vi "svx_Continuous Broadband Waveform.vi"(5 "signal type":T1(ring)=enum."Uniform white noise", 6 "sampling info":cluster{"Fs":dbl, "#s":dbl}={"Fs"=1000.0, "#s"=1000.0} {"Fs" format="%.2p"}, 7 "generation control":T2(ring), 8 "error in":errorcluster, 9 "delay until transition (0 samples)":i32, 10 "initial waveform state":cluster{"amplitude":dbl, "offset":dbl, "tf":dbl} {"tf" format="%.2f"; "offset" format="%.2f"; "amplitude" format="%.2f"}, 11 "desired waveform state":T3={"amplitude"=1.0, "offset"=0.0, "tf (ignored)"=0.0} {"tf (ignored)" format="%.2f"; "offset" format="%.2p"; "amplitude" format="%.2p"}) -> (0 "error out":errorcluster, 1 "index of transition":i32, 2 "final waveform state":cluster{"amplitude":dbl, "offset":dbl, "tf":dbl} {"tf" format="%.2f"; "offset" format="%.2f"; "amplitude" format="%.2f"}, 3 "signal out":waveform(dbl))   [LabVIEW 2017]
uses:
  <vilib>/Analysis/baseanly.llb/Inverse f Filter (DBL).vi
  <vilib>/Analysis/NI_AALBase.lvlib
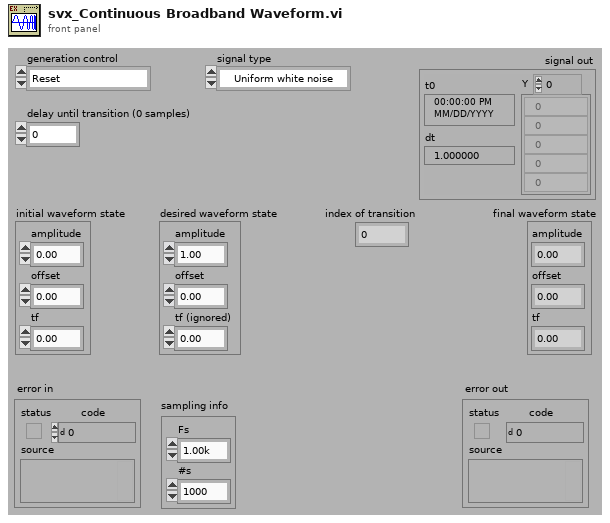
[diagram p1: front panel]
types:
  T1 = enum16{"Sine wave", "Dual tone (IMD)", "Multitone", "Chirp", "Frequency flat chirp", "Uniform white noise", "Gaussian white noise", "Pink noise", "PRN"}
  T2 = enum16{"Reset", "Continue from previous", "Continue from state", "Zero from previous", "Zero from state"}
  T3 = cluster{"amplitude":dbl, "offset":dbl, "tf (ignored)":dbl}
  T4 = cluster{"lower cutoff freq":dbl, dbl, "order":i32}
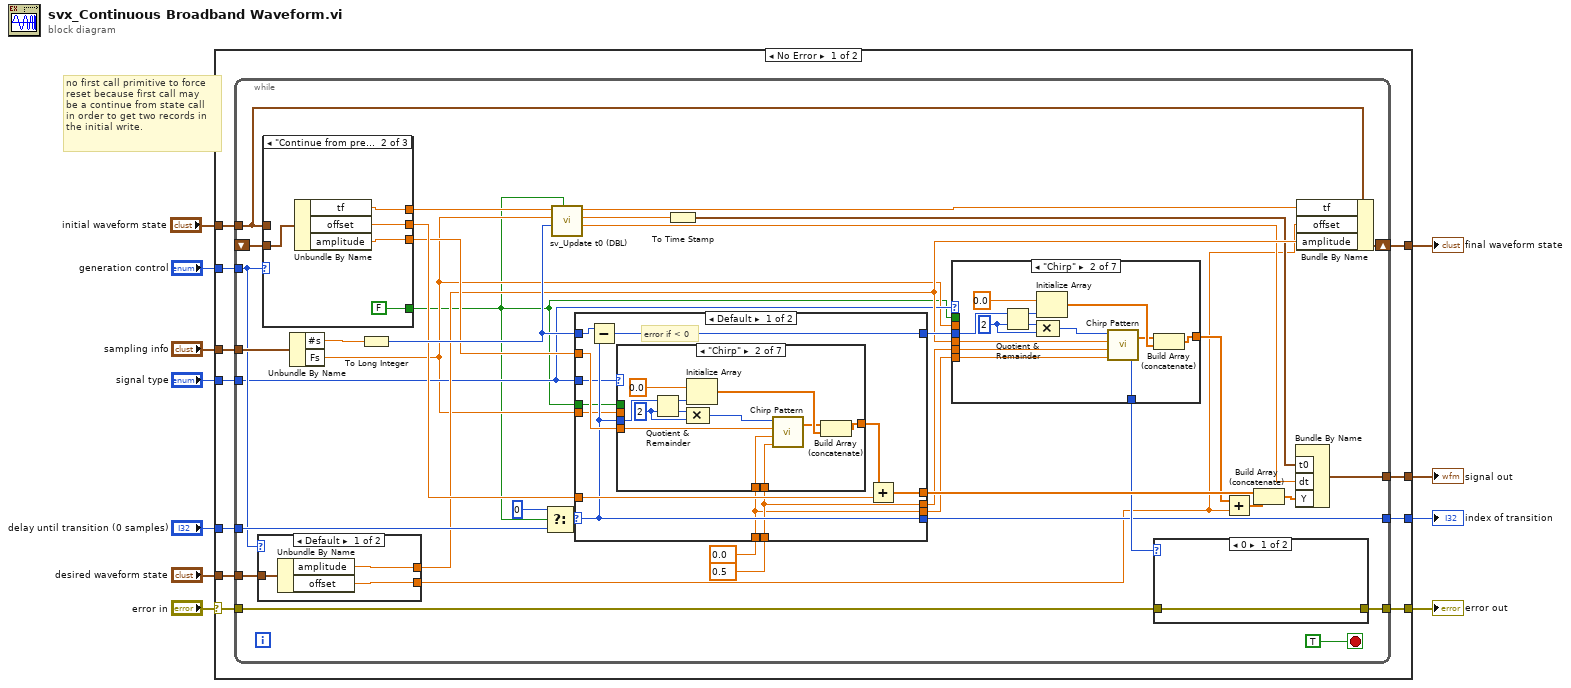
[diagram p0: block diagram]
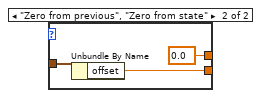
[diagram p2: hidden frame]
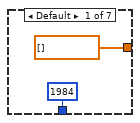
[diagram p3: hidden frame]
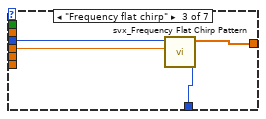
[diagram p4: hidden frame]
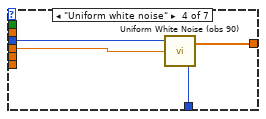
[diagram p5: hidden frame]
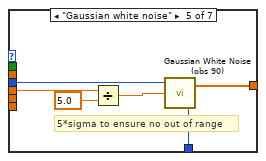
[diagram p6: hidden frame]
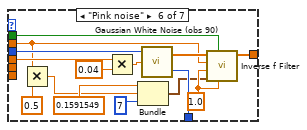
[diagram p7: hidden frame]
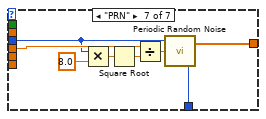
[diagram p8: hidden frame]
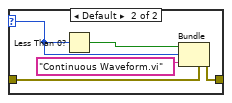
[diagram p9: hidden frame]
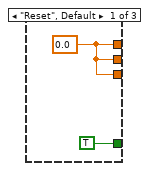
[diagram p10: hidden frame]
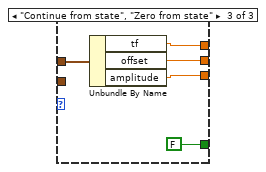
[diagram p11: hidden frame]
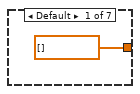
[diagram p12: hidden frame]
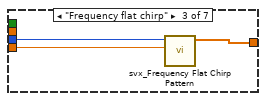
[diagram p13: hidden frame]
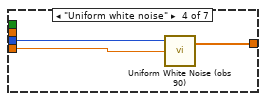
[diagram p14: hidden frame]
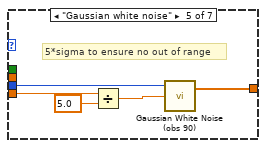
[diagram p15: hidden frame]
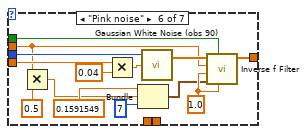
[diagram p16: hidden frame]
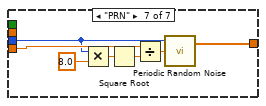
[diagram p17: hidden frame]
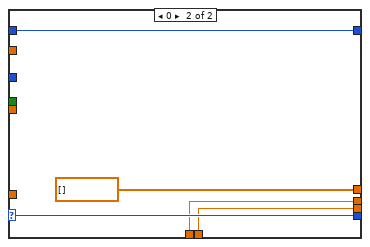
[diagram p18: hidden frame]
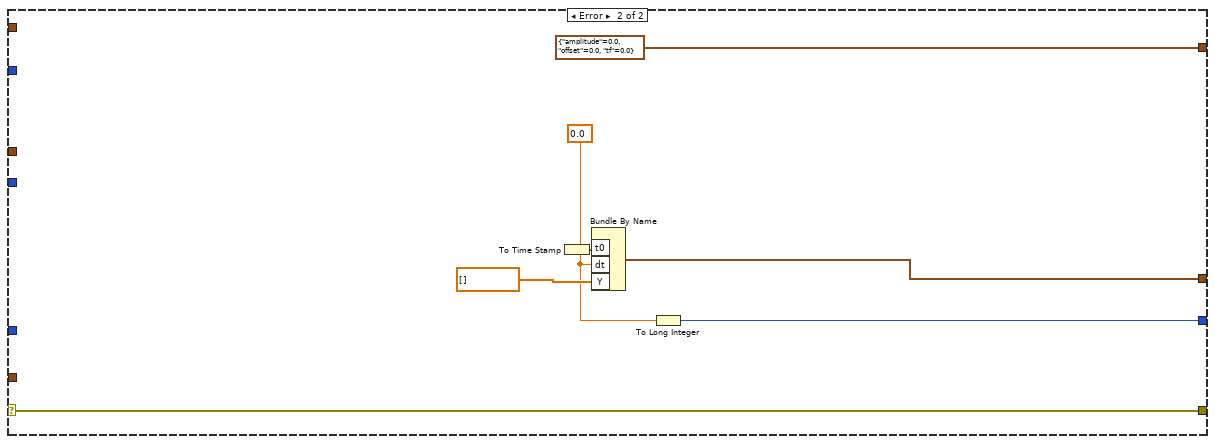
[diagram p19: hidden frame]
diagram:
  # "no first call primitive to force \nreset because first call may \nbe a continue from state call\nin order to get two records in \nthe initial write."
  n1 = case shown="No Error" "error in" {
    selector: "error in" -> [w19 w204]
    tunnel: [w21 w204] -> w10
    tunnel: [w20 w205] -> w1
    tunnel: [w18 w201] -> w9
    tunnel: "delay until transition (0 samples)" -> [w17 _]
    tunnel: [w16 cluster{"amplitude":dbl, "offset":dbl, "tf":dbl} {"amplitude"=0.0, "offset"=0.0, "tf"=0.0} ("initial waveform state")] -> w7
    tunnel: "generation control" -> [w15 _]
    tunnel: "desired waveform state" -> [w14 _]
    tunnel: "initial waveform state" -> [w13 _]
    tunnel: "signal type" -> [w12 _]
    tunnel: "sampling info" -> [w22 _]
    frame No Error {
      n2 = while {
        tunnel: w13 -> [w47]
        tunnel: w14 -> [w49]
        tunnel: w15 -> [w35]
        shift-left: _ -> [w53]
        shift-right: [w42] -> w16
        tunnel: w17 -> [w39]
        tunnel: [w31] -> w18
        tunnel: w19 -> [w45]
        tunnel: [w58] -> w20
        tunnel: [w44] -> w21
        tunnel: w12 -> [w33]
        tunnel: w22 -> [w59]
        stop <- TRUE stop-if-true
        n3 = case shown="Default" w35 {
          tunnel: w49 -> [w63 w65]
          tunnel: [w62 w64] -> w23
          tunnel: [w61 0.0 ("amplitude")] -> w34
          frame Default {
            n4 = Unbundle By Name(w63) -> ("amplitude"=w61:dbl, "offset"=w62:dbl)
          }
          frame "Zero from previous", "Zero from state" {
            n5 = Unbundle By Name(w65) -> ("offset"=w64:dbl)
          }
        }
        n6 = case shown="\"Continue from previous\", \"Zero from previous\"" w35 {
          tunnel: w53 -> [_ w130 _]
          tunnel: [TRUE FALSE FALSE] -> w25
          tunnel: [w125 w128 w134] -> w52
          tunnel: [w125 w129 w135] -> w46
          tunnel: w47 -> [_ _ w133]
          tunnel: [w125 w127 w132] -> w43
          frame "Reset", Default {
            w125 = 0.0
          }
          frame "Continue from previous", "Zero from previous" {
            n7 = Unbundle By Name(w130) -> ("tf"=w128:dbl, "offset"=w129:dbl, "amplitude"=w127:dbl)
          }
          frame "Continue from state", "Zero from state" {
            n8 = Unbundle By Name(w133) -> ("tf"=w134:dbl, "offset"=w135:dbl, "amplitude"=w132:dbl)
          }
        }
        n9 = Unbundle By Name(w59) -> ("#s"=w48:dbl, "Fs"=w32:dbl)
        n10 = To Long Integer(number=w48) -> (32bit integer=w50:i32)
        n11 = Select(t=0, s=w25, f=w39) -> (s? t:f=w38:i32)
        n12 = call <vilib>:"sv_Update t0 (DBL).vi"("Reset Generation"=w25, "samples"=w50, "sample rate (S/s)"=w32, "tf previous"=w52) -> ("dt"=w26:dbl, "t0"=w51:dbl, "tf new"=w54:dbl)  [unwired: 5 in]
        n13 = case shown="Default" w38 {
          selector: w38 -> [w142 w196]
          tunnel: w50 -> [w146 w197]
          tunnel: [w142 w196] -> w31
          tunnel: [w147 dbl[] [] ("Sine Wave")] -> w57
          tunnel: [w148 w197] -> w41
          tunnel: w46 -> [w145 _]
          tunnel: w43 -> [w143 _]
          tunnel: w33 -> [w139 _]
          tunnel: w25 -> [w140 _]
          tunnel: w32 -> [w141 _]
          tunnel: 0.0 ("f1") -> [w137 w195]
          tunnel: 0.5 ("f2") -> [w138 w194]
          tunnel: [w138 w195] -> w28
          tunnel: [w137 w194] -> w27
          frame Default {
            # "error if < 0"
            n14 = Subtract(x=w146, y=w142) -> (x-y=w148:i32)
            n15 = case shown="\"Chirp\"" w139 {
              tunnel: w142 -> [_ w157 w163 w167 w172 w182 w187]
              tunnel: w143 -> [_ w160 w164 w166 w169 w176 w192]
              tunnel: [dbl[] [] ("Periodic Random Noise") w152 w162 w165 w171 w184 w193] -> w144
              tunnel: w140 -> [_ _ _ _ _ w183 _]
              tunnel: w141 -> [_ _ _ _ _ w175 _]
              tunnel: w137 -> [_ w150 _ _ _ _ _]
              tunnel: w138 -> [_ w151 _ _ _ _ _]
              frame Default {
              }
              frame "Chirp" {
                w158 = 2 ("y")
                n16 = Quotient & Remainder(x=w157, y=w158) -> (x-y*floor(x/y)=w155:i32, floor(x/y)=w159:i32)
                n17 = Initialize Array(0.0 ("element"), w155) -> (w161:dbl[])
                n18 = Compound Arithmetic op=MULTIPLY(w159, w158) -> (w156:i32)
                n19 = call <vilib>:"Chirp Pattern.vi"("f2"=w151, "f1"=w150, "amplitude"=w160, "samples"=w156) -> ("Chirp Pattern"=w153:dbl[])  [unwired: 1 out]
                n20 = Build Array (concatenate)(w153, w161) -> (w152:dbl[])
              }
              frame "Frequency flat chirp" {
                n21 = call <vilib>:"svx_Frequency Flat Chirp Pattern.vi"("amplitude"=w164, "samples"=w163) -> ("frequency flat chirp"=w162:dbl[])  [unwired: 8 in, 1 out]
              }
              frame "Uniform white noise" {
                n22 = call <vilib>:"Uniform White Noise (obs 90).vi"("amplitude"=w166, "samples"=w167) -> ("uniform white noise"=w165:dbl[])  [unwired: 1 in, 1 out]
              }
              frame "Gaussian white noise" {
                # "5*sigma to ensure no out of range"
                n23 = Divide(x=w169, y=5.0) -> (x/y=w168:dbl)
                n24 = call <vilib>:"Gaussian White Noise (obs 90).vi"("standard deviation"=w168, "samples"=w172) -> ("Gaussian noise pattern"=w171:dbl[])  [unwired: 1 in, 1 out]
              }
              frame "Pink noise" {
                w181 = 1.0 ("exponent")
                n25 = Multiply(x=w175, y=0.5) -> (x*y=w174:dbl)
                n26 = Multiply(x=w176, y=0.04) -> (x*y=w177:dbl)
                n27 = Bundle("lower cutoff freq"=0.1591549, w174, "order"=7) -> (w180:T4)  [unwired: 1 in]
                n28 = call <vilib>:"Gaussian White Noise (obs 90).vi"("standard deviation"=w177, "samples"=w182) -> ("Gaussian noise pattern"=w186:dbl[])  [unwired: 1 in, 1 out]
                n29 = call-poly <vilib>:"Inverse f Filter.vi"("unity gain freq (rad/s)"=w181, "reset"=w183, "filter specifications"=w180, "exponent"=w181, "fs"=w175, "X"=w186) -> ("Filtered X"=w184:dbl[])  [unwired: 1 in, 4 out]
              }
              frame "PRN" {
                n30 = Multiply(x=w187, y=8.0) -> (x*y=w189:dbl)
                n31 = Square Root(x=w189) -> (sqrt(x)=w190:dbl)
                n32 = Divide(x=w192, y=w190) -> (x/y=w191:dbl)
                n33 = call <vilib>:"Periodic Random Noise.vi"("spectral amplitude"=w191, "samples"=w187) -> ("periodic random noise"=w193:dbl[])  [unwired: 1 in, 1 out]
              }
            }
            n34 = Add(x=w144, y=w145) -> (x+y=w147:dbl[])
          }
          frame 0 {
          }
        }
        n35 = To Time Stamp(1:w51) -> (0:w24:timestamp)
        n36 = case shown="\"Chirp\"" w33 {
          tunnel: w41 -> [_ w72 w84 w89 w95 w106 w111]
          tunnel: w34 -> [_ w81 w85 w88 w91 w99 w116]
          tunnel: [dbl[] [] ("Periodic Random Noise") w73 w83 w87 w94 w108 w118] -> w37
          tunnel: [1984 ("error") w80 w82 w86 w93 w104 w117] -> w36
          tunnel: w25 -> [_ _ _ _ _ w107 _]
          tunnel: w32 -> [_ _ _ _ _ w98 _]
          tunnel: w28 -> [_ w70 _ _ _ _ _]
          tunnel: w27 -> [_ w69 _ _ _ _ _]
          frame Default {
          }
          frame "Chirp" {
            w76 = 2 ("y")
            n37 = Quotient & Remainder(x=w72, y=w76) -> (x-y*floor(x/y)=w78:i32, floor(x/y)=w79:i32)
            n38 = Initialize Array(0.0 ("element"), w78) -> (w75:dbl[])
            n39 = Compound Arithmetic op=MULTIPLY(w79, w76) -> (w71:i32)
            n40 = call <vilib>:"Chirp Pattern.vi"("f2"=w69, "f1"=w70, "amplitude"=w81, "samples"=w71) -> ("error"=w80:i32, "Chirp Pattern"=w74:dbl[])
            n41 = Build Array (concatenate)(w74, w75) -> (w73:dbl[])
          }
          frame "Frequency flat chirp" {
            n42 = call <vilib>:"svx_Frequency Flat Chirp Pattern.vi"("amplitude"=w85, "samples"=w84) -> ("error"=w82:i32, "frequency flat chirp"=w83:dbl[])  [unwired: 8 in]
          }
          frame "Uniform white noise" {
            n43 = call <vilib>:"Uniform White Noise (obs 90).vi"("amplitude"=w88, "samples"=w89) -> ("error"=w86:i32, "uniform white noise"=w87:dbl[])  [unwired: 1 in]
          }
          frame "Gaussian white noise" {
            # "5*sigma to ensure no out of range"
            n44 = Divide(x=w91, y=5.0) -> (x/y=w90:dbl)
            n45 = call <vilib>:"Gaussian White Noise (obs 90).vi"("standard deviation"=w90, "samples"=w95) -> ("error"=w93:i32, "Gaussian noise pattern"=w94:dbl[])  [unwired: 1 in]
          }
          frame "Pink noise" {
            w105 = 1.0 ("exponent")
            n46 = Multiply(x=w98, y=0.5) -> (x*y=w97:dbl)
            n47 = Multiply(x=w99, y=0.04) -> (x*y=w100:dbl)
            n48 = Bundle("lower cutoff freq"=0.1591549, w97, "order"=7) -> (w103:T4)  [unwired: 1 in]
            n49 = call <vilib>:"Gaussian White Noise (obs 90).vi"("standard deviation"=w100, "samples"=w106) -> ("error"=w104:i32, "Gaussian noise pattern"=w110:dbl[])  [unwired: 1 in]
            n50 = call-poly <vilib>:"Inverse f Filter.vi"("unity gain freq (rad/s)"=w105, "reset"=w107, "filter specifications"=w103, "exponent"=w105, "fs"=w98, "X"=w110) -> ("Filtered X"=w108:dbl[])  [unwired: 1 in, 4 out]
          }
          frame "PRN" {
            n51 = Multiply(x=w111, y=8.0) -> (x*y=w113:dbl)
            n52 = Square Root(x=w113) -> (sqrt(x)=w114:dbl)
            n53 = Divide(x=w116, y=w114) -> (x/y=w115:dbl)
            n54 = call <vilib>:"Periodic Random Noise.vi"("spectral amplitude"=w115, "samples"=w111) -> ("error"=w117:i32, "periodic random noise"=w118:dbl[])  [unwired: 1 in]
          }
        }
        n55 = case shown="0" w36 {
          selector: w36 -> [_ w123]
          tunnel: w45 -> [w119 w124]
          tunnel: [w119 w120] -> w44
          frame 0 {
          }
          frame Default {
            n56 = Less Than 0?(x=w123) -> (x < 0?=w122:bool)
            n57 = Bundle(cluster=w124, "status"=w122, "code"=w123, "source"="Continuous Waveform.vi" ("subVI Name")) -> (w120:errorcluster)
          }
        }
        n58 = Add(x=w37, y=w23) -> (x+y=w56:dbl[])
        n59 = Build Array (concatenate)(w57, w56) -> (w55:dbl[])
        n60 = Bundle By Name("t0"=w24, "dt"=w26, "Y"=w55) -> (w58:waveform(dbl))  [unwired: 1 in]
        n61 = Bundle By Name(cluster=w47, "tf"=w54, "offset"=w23, "amplitude"=w34) -> (w42:cluster{"amplitude":dbl, "offset":dbl, "tf":dbl})
      }
    }
    frame Error {
      w202 = 0.0 ("t0")
      n62 = To Time Stamp(1:w202) -> (0:w199:timestamp)
      n63 = Bundle By Name("t0"=w199, "dt"=w202, "Y"=dbl[] []) -> (w205:waveform(dbl))  [unwired: 1 in]
      n64 = To Long Integer(number=w202) -> (32bit integer=w201:i32)
    }
  }
  "error out" <- w10
  "signal out" <- w1
  "index of transition" <- w9
  "final waveform state" <- w7
